vi "read timeout.vi"(8 "error in (no error)":errorcluster, 11 "Redis TCP Client in":refnum<class "Redis TCP Client.lvclass">) -> (0 "error out":errorcluster, 2 "timeout ms":i32, 3 "Redis TCP Client out":refnum<class "Redis TCP Client.lvclass">)   [LabVIEW 2019, in "Redis Client for LabVIEW.lvlib" / "Redis TCP Client.lvclass"]
uses:
  Redis TCP Client.lvclass
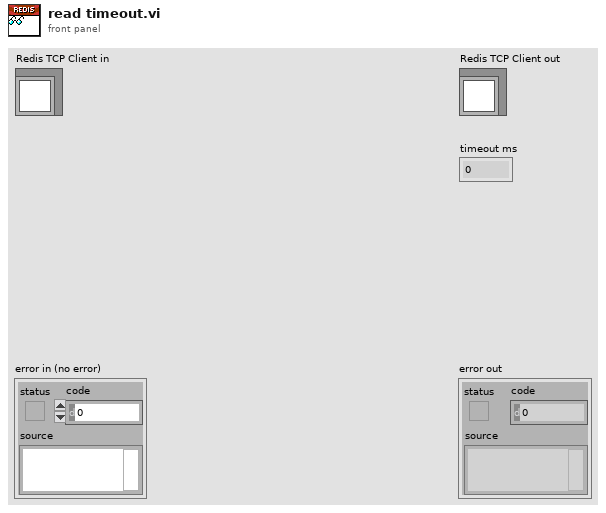
[diagram p1: front panel]
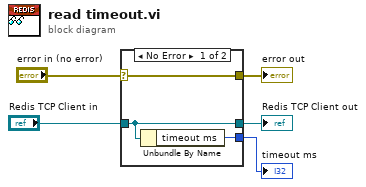
[diagram p0: block diagram]
diagram:
  n1 = case shown="No Error" "error in (no error)" {
    selector: "error in (no error)" -> [w8 w9]
    tunnel: [w8 w9] -> w4
    tunnel: [w7 w10] -> w2
    tunnel: "Redis TCP Client in" -> [w7 w10]
    tunnel: [w6 _] -> w1
    frame No Error {
      n2 = Unbundle By Name(w7) -> ("timeout ms"=w6:i32)
    }
    frame Error {
    }
  }
  "error out" <- w4
  "Redis TCP Client out" <- w2
  "timeout ms" <- w1
